vi "19_1b.vi"() -> ()   [LabVIEW 2018]
uses:
  <vilib>/regexp/Match Regular Expression.xnode
panel:
  out "sum":i16
  out "String":string
  out "element":string
  out "Rules":string[](array[string])
  out "Messages":string[](array[string])
  in  "Input":string
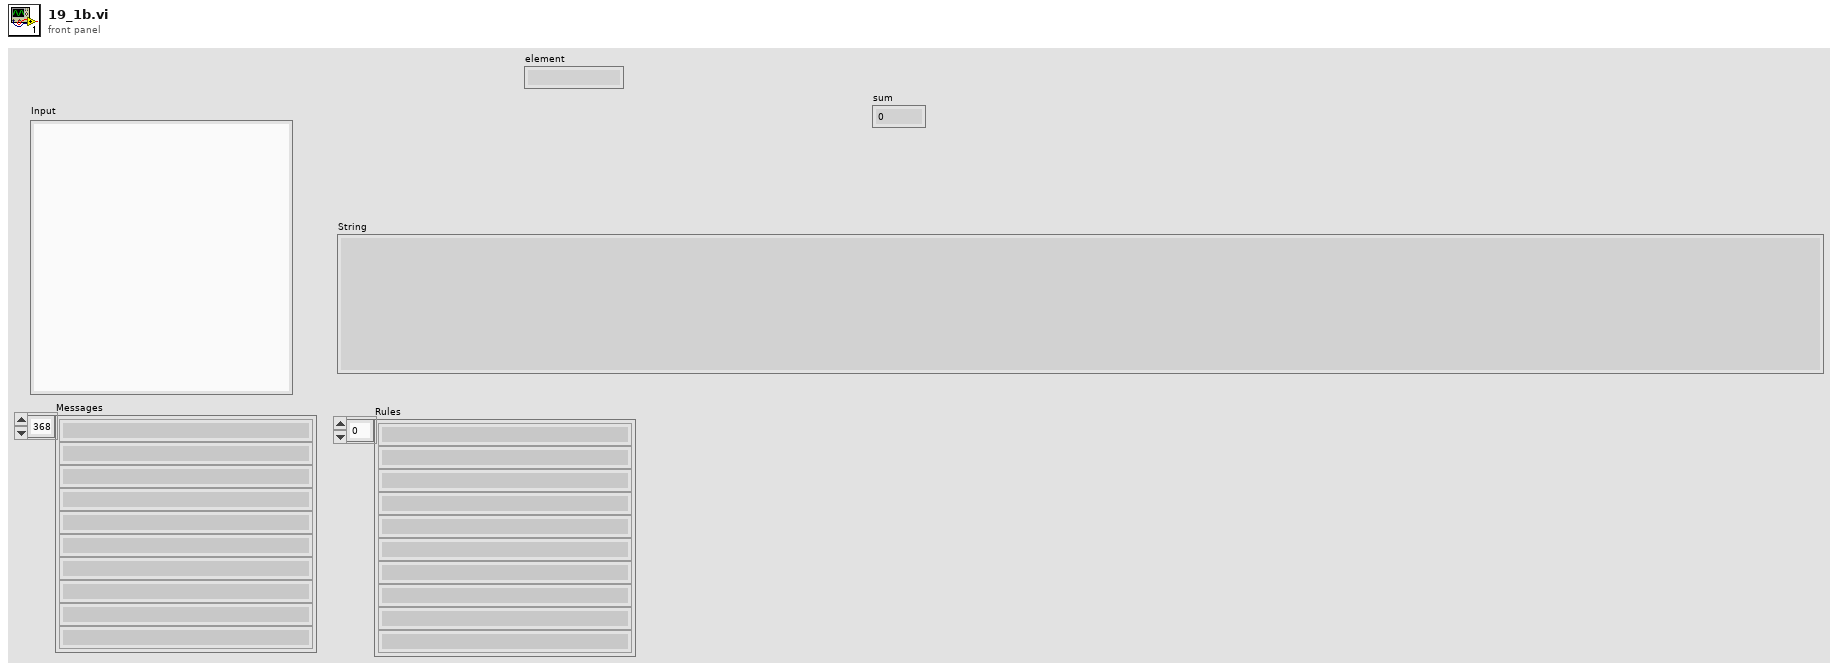
[diagram p1: front panel]
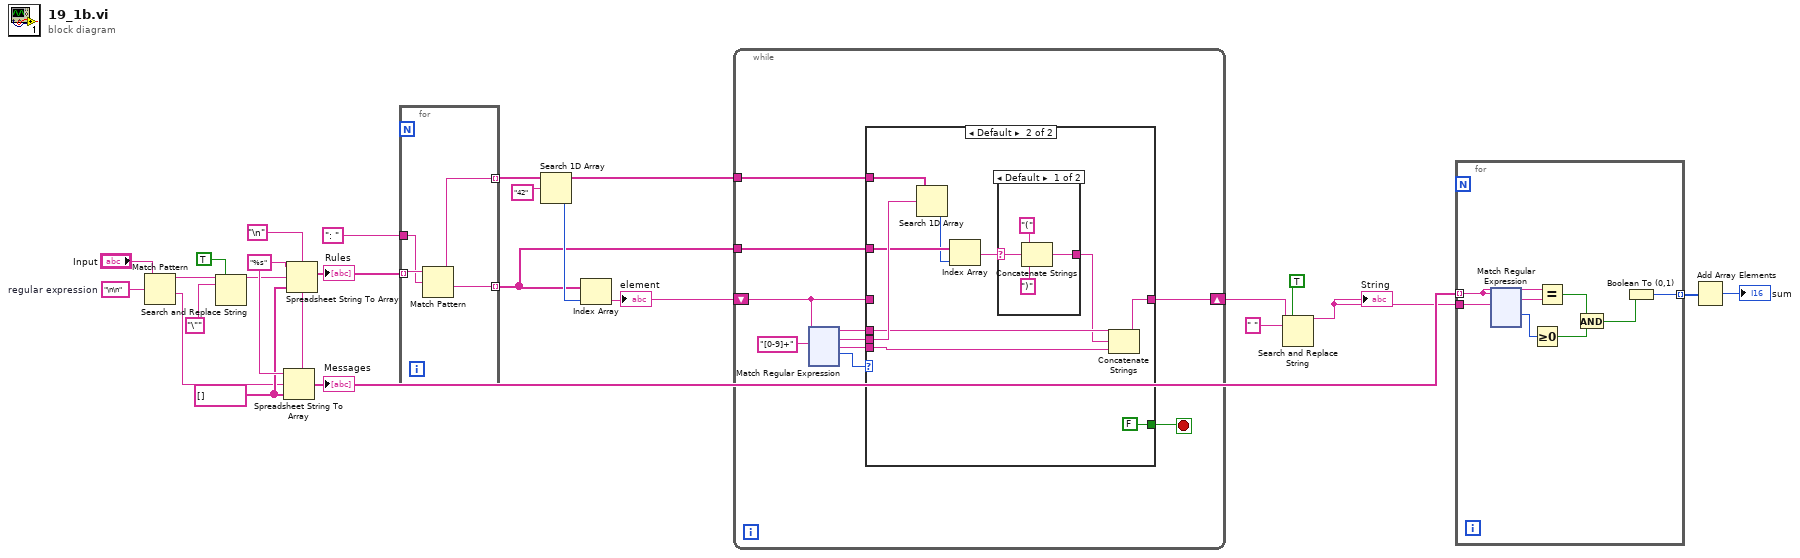
[diagram p0: block diagram]
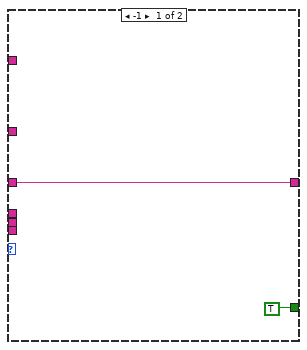
[diagram p2: hidden frame]
diagram:
  w20 = "\n"
  w22 = "%s"
  w21 = string[] []
  w23 = "\n\n"  # regular expression
  n1 = Match Pattern(string="Input", regular expression=w23) -> (before substring=w16:string, after substring=w17:string)  [unwired: 1 in, 2 out]
  n2 = Search and Replace String(replace all?=TRUE ("replace all? (F)"), input string=w16, search string="\"") -> (result string=w15:string)  [unwired: 5 in, 3 out]
  n3 = Spreadsheet String To Array(delimiter (Tab)=w20, format string=w22, spreadsheet string=w17, array type (2D Dbl)=w21) -> (array=w7:string[])
  "Messages" <- w7
  n4 = Spreadsheet String To Array(delimiter (Tab)=w20, format string=w22, spreadsheet string=w15, array type (2D Dbl)=w21) -> (array=w19:string[])
  "Rules" <- w19
  n5 = for {
    tunnel: w19 -> [w28] mode=indexing
    tunnel: ": " -> [w26]
    tunnel: [w27] -> w9 mode=indexing
    tunnel: [w25] -> w8 mode=indexing
    n6 = Match Pattern(string=w28, regular expression=w26) -> (before substring=w27:string, after substring=w25:string)  [unwired: 1 in, 2 out]
  }
  n7 = Search 1D Array(1D array=w9, element="42") -> (index of element=w11:i32)  [unwired: 1 in]
  n8 = Index Array(array=w8, index=w11) -> (element=w10:string)
  "element" <- w10
  n9 = while {
    shift-right: [w32] -> w4
    shift-left: w10 -> [w30]
    tunnel: w9 -> [w37]
    tunnel: w8 -> [w35]
    stop <- w29 stop-if-true
    n10 = xnode "Match Regular Expression"("input string"=w30, "regular expression"="[0-9]+") -> ("before match"=w34:string, "whole match"=w36:string, "after match"=w33:string, "offset past match"=w31:i32)  [unwired: 4 in, 1 out]
    n11 = case shown="Default" w31 {
      tunnel: w37 -> [_ w50]
      tunnel: w36 -> [_ w49]
      tunnel: w35 -> [_ w48]
      tunnel: w34 -> [_ w46]
      tunnel: w33 -> [_ w45]
      tunnel: [w40 w44] -> w32
      tunnel: w30 -> [w40 _]
      tunnel: [TRUE FALSE] -> w29
      frame -1 {
      }
      frame Default {
        n12 = Search 1D Array(1D array=w50, element=w49) -> (index of element=w47:i32)  [unwired: 1 in]
        n13 = Index Array(array=w48, index=w47) -> (element=w42:string)
        n14 = case shown="Default" w42 {
          selector: w42 -> [w54 w55]
          tunnel: [w53 w55] -> w41
          frame Default {
            n15 = Concatenate Strings("(", w54, ")") -> (w53:string)
          }
          frame "a", "b" {
          }
        }
        n16 = Concatenate Strings(w46, w41, w45) -> (w44:string)
      }
    }
  }
  n17 = Search and Replace String(replace all?=TRUE, input string=w4, search string=" ") -> (result string=w3:string)  [unwired: 5 in, 3 out]
  "String" <- w3
  n18 = for {
    tunnel: w3 -> [w177]
    tunnel: w7 -> [w175] mode=indexing
    tunnel: [w174] -> w6 mode=indexing
    n19 = xnode "Match Regular Expression"("input string"=w175, "regular expression"=w177) -> ("whole match"=w176:string, "offset past match"=w173:i32)  [unwired: 4 in, 3 out]
    n20 = Greater Or Equal To 0?(x=w173) -> (x >= 0?=w172:bool)
    n21 = Equal?(x=w175, y=w176) -> (x = y?=w171:bool)
    n22 = And(x=w171, y=w172) -> (x .and. y?=w170:bool)
    n23 = Boolean To (0,1)(Boolean=w170) -> (0, 1=w174:i16)
  }
  n24 = Add Array Elements(numeric array=w6) -> (sum=→"sum":i16)
